vi "Get Processes Queue Names.vi"(8 "Error In":errorcluster, 11 "Central Message Handler In":refnum<class "Central Message Handler.lvclass">) -> (0 "Error Out":errorcluster, 2 "Processes Queue Names":T1, 3 "Central Message Handler Out":refnum<class "Central Message Handler.lvclass">)   [LabVIEW 2019, in "Central Message Handler.lvclass"]
uses:
  Central Message Handler.lvclass
  Private/Controls/Processes Queue Names.ctl
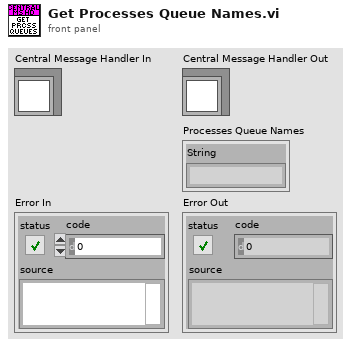
[diagram p1: front panel]
types:
  T1 = typedef "Central Message Handler.lvclass/Processes Queue Names.ctl" = cluster{"String":string}
  T2 = typedef "Central Message Handler.lvclass/Data.ctl" = cluster{"Central Message Queue":refnum<queue>, "Processes Queue Names":T1}
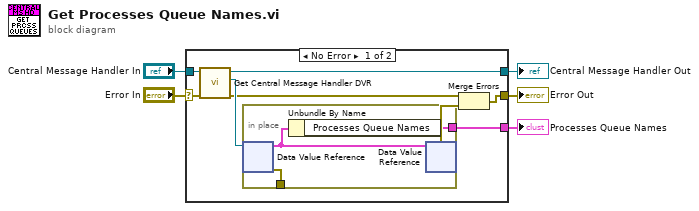
[diagram p0: block diagram]
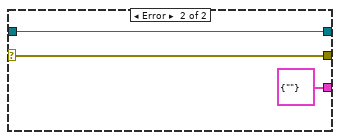
[diagram p2: hidden frame]
diagram:
  n1 = case shown="No Error" "Error In" {
    selector: "Error In" -> [w9 w18]
    tunnel: [w11 w18] -> w2
    tunnel: [w8 w19] -> w4
    tunnel: "Central Message Handler In" -> [w10 w19]
    tunnel: [w12 T1 {"String"=""} ("Processes Queue Names")] -> w1
    frame No Error {
      n2 = call "Get Central Message Handler DVR.vi"("Error In"=w9, "Central Message Handler In"=w10) -> ("Error Out"=w6:errorcluster, "DVR"=w7:refnum<data-value>, "Central Message Handler Out"=w8:refnum<class "Central Message Handler.lvclass">)  [unwired: 7 in]
      n3 = in-place {
        in-place-border: [w14] -> w12
        in-place-border: [w16] -> _
        n4 = in-place-dvr #1(w7) -> (w15:T2, w16:errorcluster)
        n5 = Unbundle By Name(w15) -> ("Processes Queue Names"=w14:T1)
        n6 = in-place-dvr #1(w15) -> (w13:errorcluster)  [unwired: 1 out]
      }
      n7 = Merge Errors(w6, w13) -> (w11:errorcluster)
    }
    frame Error {
    }
  }
  "Central Message Handler Out" <- w4
  "Error Out" <- w2
  "Processes Queue Names" <- w1
